vi "Assert Scalar wired to Array Type.vi"   [LabVIEW 2017]
uses:
  e21f47e4-c2b9-42bf-871b-0f90db9d398a.vi
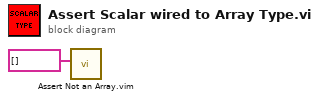
[diagram p0: block diagram]
diagram:
  n1 = call "Assert Not an Array.vim"("Input"=string[] []) -> ()  [unwired: 10 in, 1 out]
